vi "Write serial type.vi"(8 "error in (no error)":errorcluster, 10 "serial type":enum16{"RTU", "ASCII"}(ring), 11 "MiniIO in":refnum<class "MiniIO.lvclass">) -> (0 "error out":errorcluster, 3 "MiniIO out":refnum<class "MiniIO.lvclass">)   [LabVIEW 2018, in "MiniIO.lvlib" / "MiniIO.lvclass"]
uses:
  MiniIO.lvclass
  MiniIO.lvclass/MiniIO.ctl
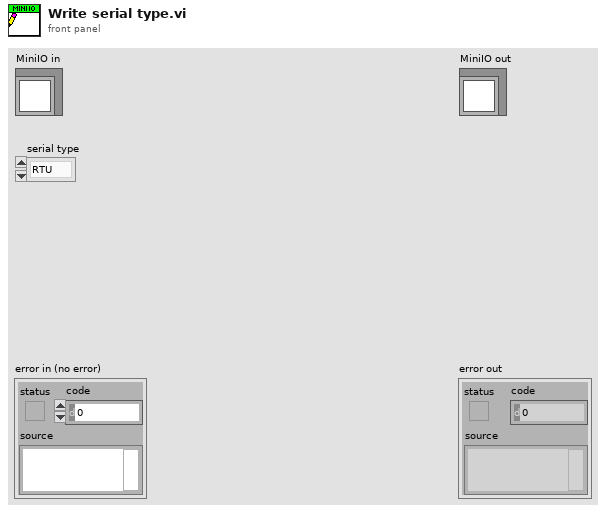
[diagram p1: front panel]
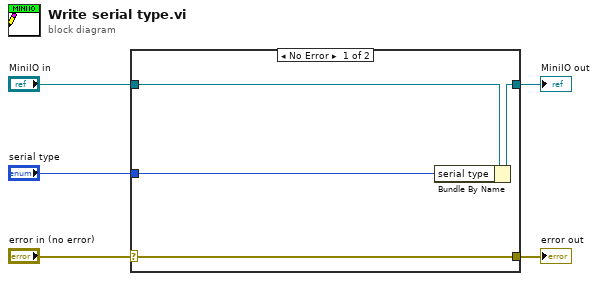
[diagram p0: block diagram]
diagram:
  n1 = case shown="No Error" "error in (no error)" {
    selector: "error in (no error)" -> [w9 w10]
    tunnel: [w9 w10] -> w4
    tunnel: [w7 w11] -> w2
    tunnel: "MiniIO in" -> [w8 w11]
    tunnel: "serial type" -> [w6 _]
    frame No Error {
      n2 = Bundle By Name(cluster=w8, "serial type"=w6) -> (w7:refnum<class "MiniIO.lvclass">)
    }
    frame Error {
    }
  }
  "error out" <- w4
  "MiniIO out" <- w2
